vi "Test Seats Occupied.vi"(11 "Error in":errorcluster) -> (15 "Error out":errorcluster)   [LabVIEW 2020, in "Airplane Tests.lvlib"]
doc: "This VI validates seat occupied tests"
uses:
  Airplane Tests.lvlib
  <vilib>/SLL Drona/APIs/Stimulus/ControlValue/SetValueAuto.vi
  <vilib>/SLL Drona/APIs/Assert/AssertControlValue/Equal.vi
  <vilib>/SLL Drona/APIs/Stimulus/VI/CloseVI.vi
  <vilib>/addons/_JKI Toolkits/Caraya/classes/Test/Test.lvclass
  <vilib>/SLL Drona/Drona.lvlib
  <vilib>/SLL Drona/APIs/Stimulus/ControlValue/ControlValue.lvlib
  <vilib>/SLL Drona/APIs/Assert/AssertControlValue/AssertControlValue.lvlib
  <vilib>/SLL Drona/APIs/Stimulus/VI/VI.lvlib
panel:
  # "SEATS OCCUPIED TEST"
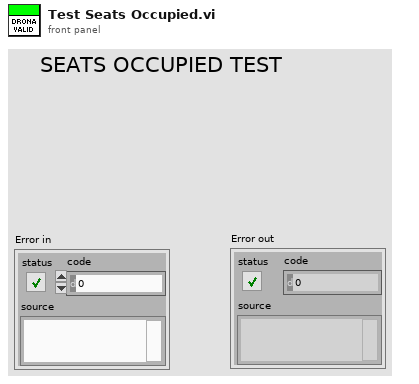
[diagram p1: front panel]
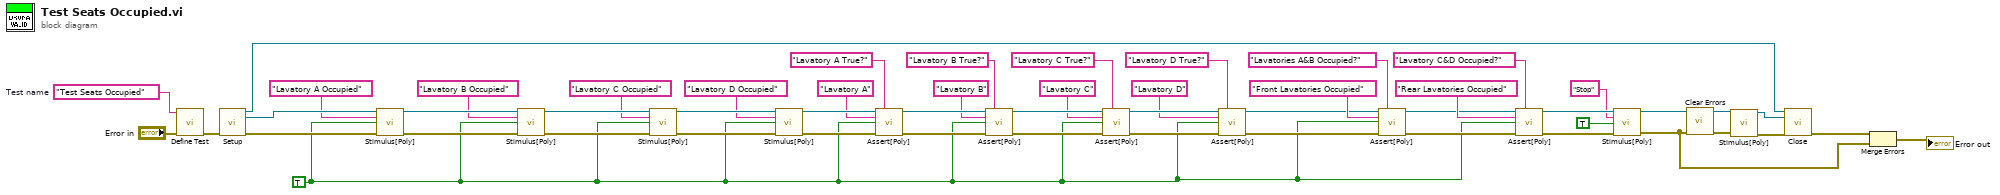
[diagram p0: block diagram]
diagram:
  w14 = TRUE
  w6 = "Test Seats Occupied"  # Test name
  n1 = call <vilib>:"Define Test.vi"("error in (no error)"="Error in", "Label (VI Title)"=w6) -> ("error out"=w52:errorcluster)  [unwired: 8 in, 1 out]
  n2 = call <vilib>:"Setup.vi"("error in"=w52) -> ("Application Ref"=w15:refnum<vi>, "VI Reference Out"=w47:refnum<vi>, "error out"=w51:errorcluster)  [unwired: 12 in]
  n3 = call-poly <vilib>:"Stimulus[Poly].vi"("VI Reference In"=w47, "Control Path"="Lavatory A Occupied", "Value (Signaling)"=w14, "error in"=w51) -> ("VI Reference Out"=w46:refnum<vi>, "error out"=w48:errorcluster)  [unwired: 10 in]
  n4 = call-poly <vilib>:"Stimulus[Poly].vi"("VI Reference In"=w46, "Control Path"="Lavatory B Occupied", "Value (Signaling)"=w14, "error in"=w48) -> ("VI Reference Out"=w45:refnum<vi>, "error out"=w50:errorcluster)  [unwired: 10 in]
  n5 = call-poly <vilib>:"Stimulus[Poly].vi"("VI Reference In"=w45, "Control Path"="Lavatory C Occupied", "Value (Signaling)"=w14, "error in"=w50) -> ("VI Reference Out"=w44:refnum<vi>, "error out"=w49:errorcluster)  [unwired: 10 in]
  n6 = call-poly <vilib>:"Stimulus[Poly].vi"("VI Reference In"=w44, "Control Path"="Lavatory D Occupied", "Value (Signaling)"=w14, "error in"=w49) -> ("VI Reference Out"=w35:refnum<vi>, "error out"=w39:errorcluster)  [unwired: 10 in]
  n7 = call-poly <vilib>:"Assert[Poly].vi"("VI Reference In"=w35, "Test Label"="Lavatory A True?" ("Control Path"), "Control Path"="Lavatory A", "Control Value"=w14, "Error In"=w39) -> ("VI Reference Out"=w34:refnum<vi>, "Error Out"=w38:errorcluster)  [unwired: 9 in]
  n8 = call-poly <vilib>:"Assert[Poly].vi"("VI Reference In"=w34, "Test Label"="Lavatory B True?" ("Control Path"), "Control Path"="Lavatory B", "Control Value"=w14, "Error In"=w38) -> ("VI Reference Out"=w33:refnum<vi>, "Error Out"=w37:errorcluster)  [unwired: 9 in]
  n9 = call-poly <vilib>:"Assert[Poly].vi"("VI Reference In"=w33, "Test Label"="Lavatory C True?" ("Control Path"), "Control Path"="Lavatory C", "Control Value"=w14, "Error In"=w37) -> ("VI Reference Out"=w32:refnum<vi>, "Error Out"=w36:errorcluster)  [unwired: 9 in]
  n10 = call-poly <vilib>:"Assert[Poly].vi"("VI Reference In"=w32, "Test Label"="Lavatory D True?" ("Control Path"), "Control Path"="Lavatory D", "Control Value"=w14, "Error In"=w36) -> ("VI Reference Out"=w17:refnum<vi>, "Error Out"=w18:errorcluster)  [unwired: 9 in]
  n11 = call-poly <vilib>:"Assert[Poly].vi"("VI Reference In"=w17, "Test Label"="Lavatories A&B Occupied?" ("Control Path"), "Control Path"="Front Lavatories Occupied", "Control Value"=w14, "Error In"=w18) -> ("VI Reference Out"=w16:refnum<vi>, "Error Out"=w23:errorcluster)  [unwired: 9 in]
  n12 = call-poly <vilib>:"Assert[Poly].vi"("VI Reference In"=w16, "Test Label"="Lavatory C&D Occupied?" ("Control Path"), "Control Path"="Rear Lavatories Occupied", "Control Value"=w14, "Error In"=w23) -> ("VI Reference Out"=w12:refnum<vi>, "Error Out"=w13:errorcluster)  [unwired: 9 in]
  n13 = call-poly <vilib>:"Stimulus[Poly].vi"("VI Reference In"=w12, "Control Path"="Stop", "Value (Signaling)"=TRUE, "error in"=w13) -> ("VI Reference Out"=w9:refnum<vi>, "error out"=w4:errorcluster)  [unwired: 10 in]
  n14 = call <vilib>:"Clear Errors.vi"("error in (no error)"=w4) -> ("error out"=w5:errorcluster)  [unwired: 5 in, 1 out]
  n15 = call-poly <vilib>:"Stimulus[Poly].vi"("VI Reference In"=w9, "error in"=w5) -> ("VI Reference Out"=w8:refnum<vi>, "error out"=w7:errorcluster)  [unwired: 12 in]
  n16 = call <vilib>:"Close.vi"("Application Ref"=w15, "VI Reference"=w8, "error in"=w7) -> ("error out"=w2:errorcluster)  [unwired: 12 in]
  n17 = Merge Errors(w2, w4) -> (→"Error out":errorcluster)
